vi "Find device name match.vi"(8 "error in":errorcluster, 10 "Saved names and data":T2[](array[typedef]), 11 "Device list":refnum<class "Device.lvclass">[](array[class])) -> (0 "error out":errorcluster, 3 "Matching pairs":T1(array[cluster]))   [LabVIEW 2015]
uses:
  Name type and data.ctl
  Device/Device type.ctl
  Device/Device.lvclass
  Device/Read Name.vi
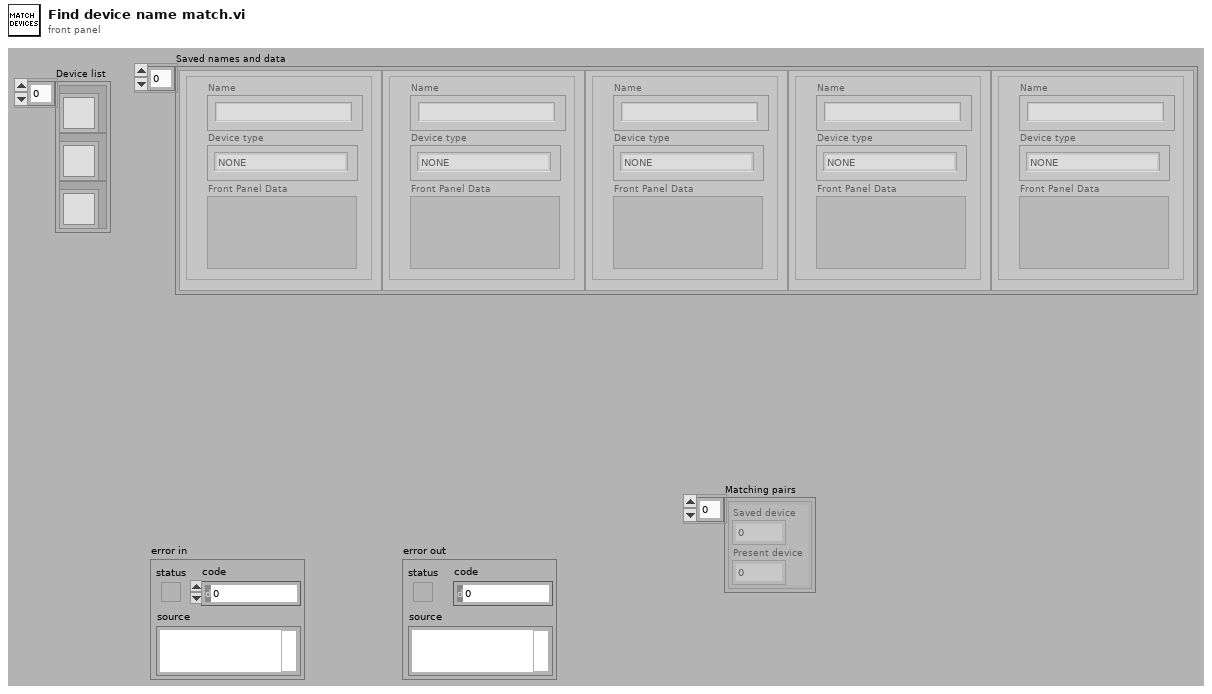
[diagram p1: front panel]
types:
  T1 = cluster{"Saved device":i32, "Present device":i32}[]
  T2 = typedef "Name type and data.ctl" = cluster{"Front Panel Data":variant, "Device type":T3, "Name":string}
  T3 = typedef "Device type.ctl" = enum16{"NONE", "Neocera 21", "LakeShore 335", "LakeShore 340", "LkShr 340 chA&B", "LakeShore 370", "SRS 850", "SRS 830", "LR 700", "EG&G 5302", "EG&G 7260", "EG&G 7280", "AH 2500", "Keithley meter", "Keithley electrometer", "Keithley 182", "HP 5385", "HP 53181", "HP 53132", "ITC503", "IPS120", "Oxford Mercury IPS", "Oxford PS", "Test", "DC Facility Magnet", "Cryomagnetics PS", "Keithley 2400", "Keithley current source", "Cryo-Con 22C", "HP87NN", "HP4395A"}
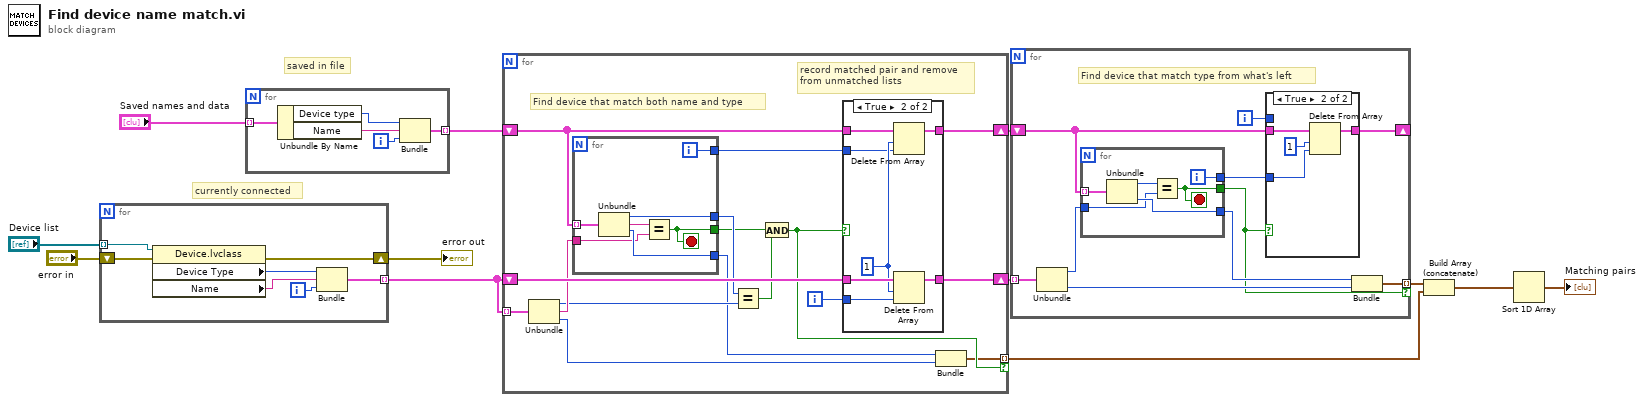
[diagram p0: block diagram]
diagram:
  # "saved in file"
  # "currently connected"
  n1 = for {
    tunnel: "Device list" -> [w19] mode=indexing
    tunnel: [w15] -> w9 mode=indexing
    shift-right: [w13] -> w5
    shift-left: "error in" -> [w14]
    i -> [w16]
    n2 = property class="Device.lvclass"(reference=w19, error in=w14) -> (error out=w13:errorcluster, "Device Type"=w18:T3, "Name"=w17:string)  [unwired: 1 out]
    n3 = Bundle("Device Type"=w18, "Name"=w17, w16) -> (w15:cluster{"Device Type":T3, "Name":string, i32})  [unwired: 1 in]
  }
  "error out" <- w5
  n4 = for {
    tunnel: "Saved names and data" -> [w24] mode=indexing
    tunnel: [w20] -> w10 mode=indexing
    i -> [w21]
    n5 = Unbundle By Name(w24) -> ("Device type"=w23:T3, "Name"=w22:string)
    n6 = Bundle("Device type"=w23, "Name"=w22, w21) -> (w20:cluster{"Device type":T3, "Name":string, i32})  [unwired: 1 in]
  }
  n7 = for {
    shift-right: [w39] -> w8
    shift-left: w9 -> [w40]
    shift-right: [w37] -> w7
    shift-left: w10 -> [w36]
    tunnel: w9 -> [w33] mode=indexing
    tunnel: [w25] -> w3 mode=indexing if=w28
    i -> [w38]
    # "Find device that match both name and type"
    # "record matched pair and remove\nfrom unmatched lists"
    n8 = Unbundle(w33) -> ("Device Type"=w32:T3, "Name"=w35:string, w26:i32)
    n9 = for {
      tunnel: w36 -> [w47] mode=indexing
      tunnel: w35 -> [w42]
      tunnel: [w46] -> w29
      tunnel: [w45] -> w34
      tunnel: [w44] -> w31
      tunnel: [w43] -> w27
      i -> [w45]
      stop <- w46 stop-if-true
      n10 = Unbundle(w47) -> ("Device type"=w44:T3, "Name"=w41:string, w43:i32)
      n11 = Equal?(x=w41, y=w42) -> (x = y?=w46:bool)
    }
    n12 = Equal?(x=w31, y=w32) -> (x = y?=w30:bool)
    n13 = And(x=w29, y=w30) -> (x .and. y?=w28:bool)
    n14 = case shown="True" w28 {
      tunnel: w40 -> [w49 w56]
      tunnel: [w49 w55] -> w39
      tunnel: w38 -> [_ w51]
      tunnel: w36 -> [w48 w54]
      tunnel: [w48 w53] -> w37
      tunnel: w34 -> [_ w50]
      frame False {
      }
      frame True {
        w52 = 1 ("length")
        n15 = Delete From Array(array=w54, length=w52, index=w50) -> (array with subset deleted=w53:cluster{"Device type":T3, "Name":string, i32}[])  [unwired: 1 out]
        n16 = Delete From Array(array=w56, length=w52, index=w51) -> (array with subset deleted=w55:cluster{"Device Type":T3, "Name":string, i32}[])  [unwired: 1 out]
      }
    }
    n17 = Bundle(w27, w26) -> (w25:cluster{i32, i32})  [unwired: 1 in]
  }
  n18 = for {
    shift-right: [w65] -> _
    shift-left: w7 -> [w64]
    tunnel: w8 -> [w62] mode=indexing
    tunnel: [w58] -> w4 mode=indexing if=w57
    i -> [w66]
    # "Find device that match type from what's left"
    n19 = Unbundle(w62) -> ("Device Type"=w61:T3, w59:i32)  [unwired: 1 out]
    n20 = for {
      tunnel: w64 -> [w72] mode=indexing
      tunnel: w61 -> [w67]
      tunnel: [w71] -> w57
      tunnel: [w70] -> w63
      tunnel: [w69] -> w60
      i -> [w70]
      stop <- w71 stop-if-true
      n21 = Unbundle(w72) -> ("Device type"=w68:T3, w69:i32)  [unwired: 1 out]
      n22 = Equal?(x=w68, y=w67) -> (x = y?=w71:bool)
    }
    n23 = case shown="True" w57 {
      tunnel: w66 -> [_ _]
      tunnel: w64 -> [w73 w77]
      tunnel: [w73 w76] -> w65
      tunnel: w63 -> [_ w74]
      frame False {
      }
      frame True {
        n24 = Delete From Array(array=w77, length=1, index=w74) -> (array with subset deleted=w76:cluster{"Device type":T3, "Name":string, i32}[])  [unwired: 1 out]
      }
    }
    n25 = Bundle(w60, w59) -> (w58:cluster{i32, i32})  [unwired: 1 in]
  }
  n26 = Build Array (concatenate)(w4, w3) -> (w2:cluster{i32, i32}[])
  n27 = Sort 1D Array(array=w2) -> (sorted array=→"Matching pairs":cluster{i32, i32}[])
